vi "Pressure Set.vi"(8 "error in":errorcluster, 9 "Val":dbl, 10 "Pressure Box COM":refnum<visa-resource-name>, 11 "arduino pressure setting":T1=enum."Low Positive Pressure") -> (0 "error out":errorcluster, 2 "Pressure Box COM out":refnum<visa-resource-name>)   [LabVIEW 2019]
uses:
  controls/arduino_pressure_setting.ctl
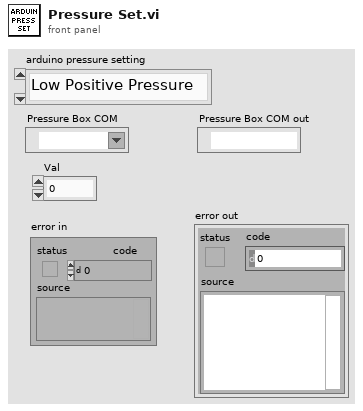
[diagram p1: front panel]
types:
  T1 = typedef "arduino_pressure_setting.ctl" = enum16{"High Positive Pressure", "Low Positive Pressure", "Atmospheric Pressure", "Low Vacuum", "High Vacuum", "Break In", "Puff"}
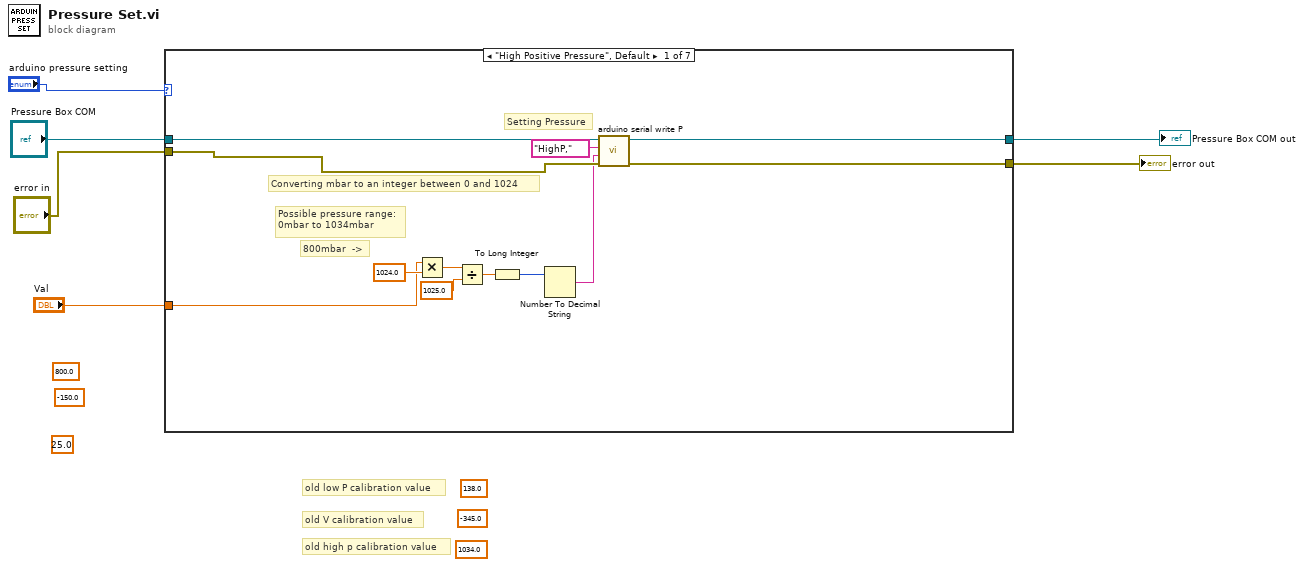
[diagram p0: block diagram]
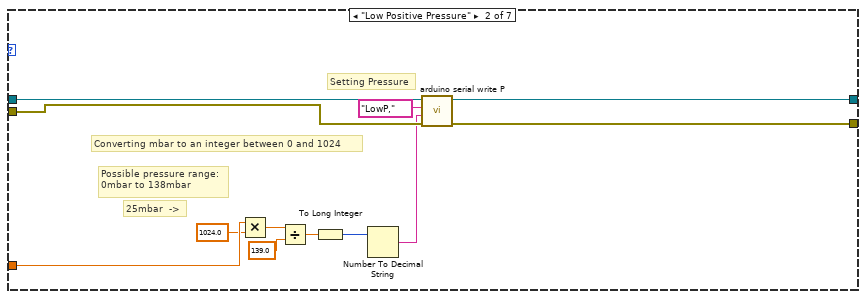
[diagram p2: hidden frame]
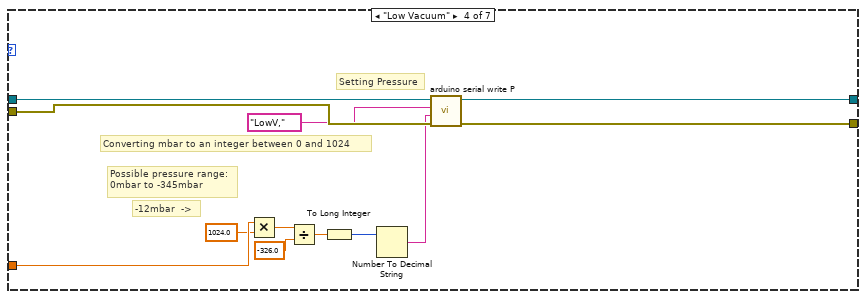
[diagram p4: hidden frame]
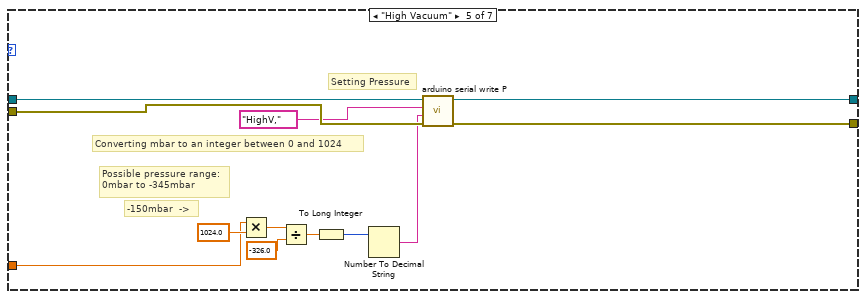
[diagram p5: hidden frame]
diagram:
  (unwired) 1034.0 ("y")
  (unwired) -345.0 ("y")
  (unwired) 138.0 ("y")
  (unwired) 25.0 ("x")
  (unwired) 800.0 ("x")
  (unwired) -150.0 ("x")
  # "old high p calibration value"
  # "old V calibration value"
  # "old low P calibration value"
  n1 = case shown="\"High Positive Pressure\", Default" "arduino pressure setting" {
    tunnel: "Pressure Box COM" -> [w18 w30 w32 w44 w56 w58 w60]
    tunnel: "error in" -> [w17 w29 w31 w43 w55 w57 w59]
    tunnel: [w8 w19 w31 w33 w46 w57 w59] -> w4
    tunnel: [w9 w20 w32 w34 w47 w58 w60] -> w3
    tunnel: "Val" -> [w7 w28 _ w42 w45 _ _]
    frame "High Positive Pressure", Default {
      # "Possible pressure range:\n0mbar to 1034mbar"
      # "Converting mbar to an integer between 0 and 1024"
      # "Setting Pressure"
      # "800mbar  ->"
      n2 = Multiply(x=w7, y=1024.0) -> (x*y=w15:dbl)
      n3 = Divide(x=w15, y=1025.0) -> (x/y=w13:dbl)
      n4 = To Long Integer(number=w13) -> (32bit integer=w11:i32)
      n5 = Number To Decimal String(number=w11) -> (decimal integer string=w12:string)  [unwired: 1 in]
      n6 = call "arduino serial write P.vi"("error in"=w17, "DAC value (0-1024)"=w12, "DAC output"="HighP,", "Pressure Box COM"=w18) -> ("error out"=w8:errorcluster, "Pressure Box COM out"=w9:refnum<visa-resource-name>)  [unwired: 6 in]
    }
    frame "Low Positive Pressure" {
      # "Possible pressure range:\n0mbar to 138mbar"
      # "Converting mbar to an integer between 0 and 1024"
      # "Setting Pressure"
      # "25mbar  ->"
      n7 = Multiply(x=w28, y=1024.0) -> (x*y=w26:dbl)
      n8 = Divide(x=w26, y=139.0) -> (x/y=w24:dbl)
      n9 = To Long Integer(number=w24) -> (32bit integer=w22:i32)
      n10 = Number To Decimal String(number=w22) -> (decimal integer string=w23:string)  [unwired: 1 in]
      n11 = call "arduino serial write P.vi"("error in"=w29, "DAC value (0-1024)"=w23, "DAC output"="LowP,", "Pressure Box COM"=w30) -> ("error out"=w19:errorcluster, "Pressure Box COM out"=w20:refnum<visa-resource-name>)  [unwired: 6 in]
    }
    frame "Atmospheric Pressure" {
    }
    frame "Low Vacuum" {
      # "Possible pressure range:\n0mbar to -345mbar"
      # "Converting mbar to an integer between 0 and 1024"
      # "Setting Pressure"
      # "-12mbar  ->"
      n12 = Multiply(x=w42, y=1024.0) -> (x*y=w40:dbl)
      n13 = Divide(x=w40, y=-326.0) -> (x/y=w38:dbl)
      n14 = To Long Integer(number=w38) -> (32bit integer=w36:i32)
      n15 = Number To Decimal String(number=w36) -> (decimal integer string=w37:string)  [unwired: 1 in]
      n16 = call "arduino serial write P.vi"("error in"=w43, "DAC value (0-1024)"=w37, "DAC output"="LowV,", "Pressure Box COM"=w44) -> ("error out"=w33:errorcluster, "Pressure Box COM out"=w34:refnum<visa-resource-name>)  [unwired: 6 in]
    }
    frame "High Vacuum" {
      # "Possible pressure range:\n0mbar to -345mbar"
      # "Converting mbar to an integer between 0 and 1024"
      # "Setting Pressure"
      # "-150mbar  ->"
      n17 = Multiply(x=w45, y=1024.0) -> (x*y=w53:dbl)
      n18 = Divide(x=w53, y=-326.0) -> (x/y=w51:dbl)
      n19 = To Long Integer(number=w51) -> (32bit integer=w49:i32)
      n20 = Number To Decimal String(number=w49) -> (decimal integer string=w50:string)  [unwired: 1 in]
      n21 = call "arduino serial write P.vi"("error in"=w55, "DAC value (0-1024)"=w50, "DAC output"="HighV,", "Pressure Box COM"=w56) -> ("error out"=w46:errorcluster, "Pressure Box COM out"=w47:refnum<visa-resource-name>)  [unwired: 6 in]
    }
    frame "Break In" {
    }
    frame "Puff" {
    }
  }
  "error out" <- w4
  "Pressure Box COM out" <- w3
